vi "Get_Temperature_Status.vi"(0 "Status Array":T1(array[cluster])) -> (1 "Setpoint":dbl, 2 "Temperature":dbl, 3 "Power":dbl)   [LabVIEW 2011]
doc: "This VI iterates through the given \"Status Array\" until it finds a temperature status, which is parses. Numerical values indicating current Setpoint (C), Temperature (C), and Power (%) are returned."
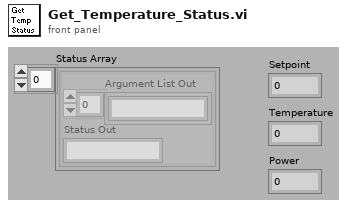
[diagram p1: front panel]
types:
  T1 = cluster{"Argument List Out":string[], "Status Out":string}[]
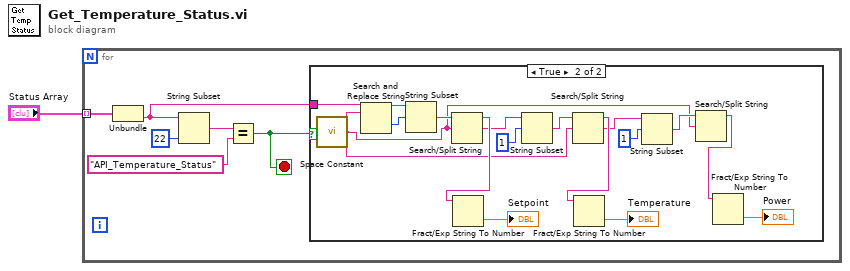
[diagram p0: block diagram]
diagram:
  n1 = for {
    tunnel: "Status Array" -> [w7] mode=indexing
    stop <- w4 stop-if-true
    n2 = Unbundle(w7) -> ("Status Out"=w2:string)  [unwired: 1 out]
    n3 = String Subset(string=w2, length (rest)=22 ("length (rest)")) -> (substring=w3:string)  [unwired: 1 out]
    n4 = Equal?(x=w3, y="API_Temperature_Status") -> (x = y?=w4:bool)
    n5 = case shown="True" w4 {
      tunnel: w2 -> [_ w24]
      frame False {
      }
      frame True {
        n6 = call <vilib>:"Space Constant.vi"() -> ("String"=w10:string)
        n7 = Search and Replace String(input string=w24, search string=w10) -> (result string=w23:string, offset past replacement=w22:i32)  [unwired: 1 in, 7 out]
        n8 = String Subset(string=w23, offset (0)=w22) -> (substring=w21:string)  [unwired: 1 out]
        n9 = Search/Split String(string=w21, search string/char (-)=w10) -> (substring before match=w19:string, match + rest of string=w18:string)  [unwired: 2 out]
        n10 = Fract/Exp String To Number(string=w19) -> (number=→"Setpoint":dbl)  [unwired: 4 out]
        n11 = String Subset(string=w18, offset (0)=1) -> (substring=w16:string)  [unwired: 1 out]
        n12 = Search/Split String(string=w16, search string/char (-)=w10) -> (substring before match=w15:string, match + rest of string=w13:string)  [unwired: 2 out]
        n13 = Fract/Exp String To Number(string=w15) -> (number=→"Temperature":dbl)  [unwired: 4 out]
        n14 = String Subset(string=w13, offset (0)=1) -> (substring=w11:string)  [unwired: 1 out]
        n15 = Search/Split String(string=w11, search string/char (-)=w10) -> (substring before match=w9:string)  [unwired: 3 out]
        n16 = Fract/Exp String To Number(string=w9) -> (number=→"Power":dbl)  [unwired: 4 out]
      }
    }
  }
